vi "sine.vi"(7 "number of x points":i32=201, 8 "amplitude":dbl=1.0, 9 "phase":dbl, 10 "frequency":dbl=10000000.0, 11 "Sampling rate":i64=2000000000 format="%.0p") -> (1 "phase out (deg)":dbl[](array[numeric])=[0.0, 1.8000000000000003, 3.6000000000000005, 5.4, 7.200000000000001, 9.000000000000002, 10.8, 12.600000000000001, 14.400000000000002, 16.200000000000003, 18.000000000000004, 19.799999999999997, 21.6, 23.400000000000002, 25.200000000000003, 27.000000000000004, 28.800000000000004, 30.599999999999998, 32.400000000000006, 34.2, 36.00000000000001, 37.8, 39.599999999999994, 41.4, 43.2, 45.0, 46.800000000000004, 48.6, 50.400000000000006, 52.2, 54.00000000000001, 55.8, 57.60000000000001, 59.40000000000001, 61.199999999999996, 63.000000000000014, 64.80000000000001, 66.60000000000001, 68.4, 70.2, 72.00000000000001, 73.80000000000003, 75.6, 77.39999999999999, 79.19999999999999, 81.0, 82.8, 84.6, 86.4, 88.2, 90.0, 91.8, 93.60000000000001, 95.4, 97.2, 99.00000000000001, 100.80000000000001, 102.60000000000001, 104.4, 106.20000000000002, 108.00000000000001, 109.8, 111.6, 113.4, 115.20000000000002, 117.0, 118.80000000000003, 120.60000000000001, 122.39999999999999, 124.2, 126.00000000000003, 127.80000000000001, 129.60000000000002, 131.40000000000003, 133.20000000000002, 135.00000000000003, 136.8, 138.6, 140.4, 142.20000000000002, 144.00000000000003, 145.8, 147.60000000000005, 149.40000000000003, 151.2, 153.0, 154.79999999999998, 156.6, 158.39999999999998, 160.20000000000002, 162.0, 163.79999999999998, 165.6, 167.4, 169.2, 171.0, 172.8, 174.6, 176.4, 178.20000000000002, 180.0, 181.8, 183.6, 185.4, 187.20000000000002, 189.0, 190.8, 192.60000000000002, 194.4, 196.20000000000002, 198.00000000000003, 199.8, 201.60000000000002, 203.4, 205.20000000000002, 207.00000000000003, 208.8, 210.6, 212.40000000000003, 214.20000000000002, 216.00000000000003, 217.80000000000004, 219.6, 221.40000000000003, 223.2, 225.00000000000003, 226.8, 228.60000000000002, 230.40000000000003, 232.2, 234.0, 235.8, 237.60000000000005, 239.4, 241.20000000000002, 243.0, 244.79999999999998, 246.59999999999997, 248.4, 250.20000000000002, 252.00000000000006, 253.79999999999998, 255.60000000000002, 257.40000000000003, 259.20000000000005, 261.0, 262.80000000000007, 264.6, 266.40000000000003, 268.20000000000005, 270.00000000000006, 271.8, 273.6, 275.40000000000003, 277.2, 279.0, 280.8, 282.6, 284.40000000000003, 286.2, 288.00000000000006, 289.8, 291.6, 293.4, 295.2000000000001, 297.0, 298.80000000000007, 300.6, 302.4, 304.2, 306.0, 307.80000000000007, 309.59999999999997, 311.40000000000003, 313.2, 315.0, 316.79999999999995, 318.6, 320.40000000000003, 322.20000000000005, 324.0, 325.8, 327.59999999999997, 329.4, 331.2, 333.00000000000006, 334.8, 336.6, 338.4, 340.2, 342.0, 343.80000000000007, 345.6, 347.4, 349.2, 351.00000000000006, 352.8, 354.6, 356.40000000000003, 358.2, 0.0], 2 "y":dbl[](array[numeric])=[0.0, 0.03141075907812829, 0.06279051952931337, 0.09410831331851431, 0.12533323356430426, 0.1564344650402309, 0.1873813145857246, 0.21814324139654254, 0.2486898871648548, 0.2789911060392293, 0.30901699437494745, 0.33873792024529137, 0.3681245526846779, 0.3971478906347806, 0.42577929156507266, 0.4539904997395468, 0.4817536741017153, 0.5090414157503712, 0.5358267949789967, 0.5620833778521306, 0.5877852522924732, 0.6129070536529764, 0.6374239897486896, 0.6613118653236518, 0.6845471059286886, 0.7071067811865476, 0.7289686274214116, 0.7501110696304596, 0.7705132427757893, 0.7901550123756904, 0.8090169943749475, 0.8270805742745618, 0.8443279255020151, 0.8607420270039436, 0.8763066800438636, 0.8910065241883679, 0.9048270524660196, 0.9177546256839811, 0.9297764858882515, 0.9408807689542256, 0.9510565162951536, 0.9602936856769432, 0.9685831611286311, 0.9759167619387473, 0.9822872507286886, 0.9876883405951378, 0.9921147013144779, 0.99556196460308, 0.9980267284282716, 0.9995065603657316, 1.0, 0.9995065603657316, 0.9980267284282716, 0.99556196460308, 0.9921147013144778, 0.9876883405951378, 0.9822872507286887, 0.9759167619387474, 0.9685831611286311, 0.9602936856769431, 0.9510565162951535, 0.9408807689542255, 0.9297764858882515, 0.9177546256839811, 0.9048270524660195, 0.8910065241883679, 0.8763066800438635, 0.8607420270039436, 0.8443279255020152, 0.8270805742745617, 0.8090169943749472, 0.7901550123756903, 0.7705132427757893, 0.7501110696304594, 0.7289686274214114, 0.7071067811865472, 0.6845471059286885, 0.6613118653236518, 0.6374239897486895, 0.6129070536529764, 0.5877852522924728, 0.5620833778521305, 0.5358267949789962, 0.5090414157503711, 0.4817536741017156, 0.45399049973954686, 0.4257792915650729, 0.3971478906347806, 0.36812455268467814, 0.3387379202452913, 0.3090169943749475, 0.27899110603922955, 0.24868988716485482, 0.21814324139654276, 0.18738131458572457, 0.15643446504023098, 0.12533323356430454, 0.09410831331851435, 0.06279051952931358, 0.031410759078128236, 1.2246467991473532e-16, -0.03141075907812844, -0.06279051952931335, -0.0941083133185141, -0.12533323356430429, -0.15643446504023073, -0.18738131458572477, -0.2181432413965425, -0.24868988716485502, -0.2789911060392293, -0.3090169943749473, -0.3387379202452915, -0.3681245526846779, -0.3971478906347808, -0.42577929156507266, -0.4539904997395471, -0.4817536741017154, -0.5090414157503712, -0.5358267949789968, -0.5620833778521306, -0.5877852522924734, -0.6129070536529766, -0.6374239897486896, -0.661311865323652, -0.6845471059286887, -0.7071067811865477, -0.7289686274214116, -0.7501110696304598, -0.7705132427757894, -0.7901550123756904, -0.8090169943749473, -0.8270805742745616, -0.8443279255020153, -0.8607420270039438, -0.8763066800438636, -0.8910065241883678, -0.9048270524660194, -0.9177546256839809, -0.9297764858882515, -0.9408807689542255, -0.9510565162951538, -0.960293685676943, -0.9685831611286312, -0.9759167619387474, -0.9822872507286887, -0.9876883405951377, -0.9921147013144779, -0.99556196460308, -0.9980267284282716, -0.9995065603657316, -1.0, -0.9995065603657316, -0.9980267284282716, -0.99556196460308, -0.9921147013144779, -0.9876883405951378, -0.9822872507286886, -0.9759167619387473, -0.9685831611286311, -0.9602936856769431, -0.9510565162951533, -0.9408807689542256, -0.9297764858882512, -0.917754625683981, -0.9048270524660191, -0.891006524188368, -0.8763066800438634, -0.8607420270039434, -0.8443279255020155, -0.8270805742745618, -0.8090169943749476, -0.7901550123756901, -0.7705132427757896, -0.7501110696304595, -0.7289686274214116, -0.7071067811865477, -0.684547105928689, -0.6613118653236516, -0.6374239897486896, -0.6129070536529765, -0.5877852522924734, -0.5620833778521301, -0.5358267949789971, -0.5090414157503712, -0.4817536741017153, -0.4539904997395462, -0.425779291565073, -0.39714789063478034, -0.36812455268467786, -0.3387379202452914, -0.3090169943749477, -0.2789911060392288, -0.24868988716485535, -0.21814324139654243, -0.18738131458572468, -0.15643446504023023, -0.12533323356430465, -0.09410831331851403, -0.06279051952931326, -0.03141075907812836, -2.4492935982947064e-16], 3 "x":dbl[](array[numeric])=[0.0, 1.0, 2.0, 3.0, 4.0, 5.0, 6.0, 7.0, 8.0, 9.0, 10.0, 11.0, 12.0, 13.0, 14.0, 15.0, 16.0, 17.0, 18.0, 19.0, 20.0, 21.0, 22.0, 23.0, 24.0, 25.0, 26.0, 27.0, 28.0, 29.0, 30.0, 31.0, 32.0, 33.0, 34.0, 35.0, 36.0, 37.0, 38.0, 39.0, 40.0, 41.0, 42.0, 43.0, 44.0, 45.0, 46.0, 47.0, 48.0, 49.0, 50.0, 51.0, 52.0, 53.0, 54.0, 55.0, 56.0, 57.0, 58.0, 59.0, 60.0, 61.0, 62.0, 63.0, 64.0, 65.0, 66.0, 67.0, 68.0, 69.0, 70.0, 71.0, 72.0, 73.0, 74.0, 75.0, 76.0, 77.0, 78.0, 79.0, 80.0, 81.0, 82.0, 83.0, 84.0, 85.0, 86.0, 87.0, 88.0, 89.0, 90.0, 91.0, 92.0, 93.0, 94.0, 95.0, 96.0, 97.0, 98.0, 99.0, 100.0, 101.0, 102.0, 103.0, 104.0, 105.0, 106.0, 107.0, 108.0, 109.0, 110.0, 111.0, 112.0, 113.0, 114.0, 115.0, 116.0, 117.0, 118.0, 119.0, 120.0, 121.0, 122.0, 123.0, 124.0, 125.0, 126.0, 127.0, 128.0, 129.0, 130.0, 131.0, 132.0, 133.0, 134.0, 135.0, 136.0, 137.0, 138.0, 139.0, 140.0, 141.0, 142.0, 143.0, 144.0, 145.0, 146.0, 147.0, 148.0, 149.0, 150.0, 151.0, 152.0, 153.0, 154.0, 155.0, 156.0, 157.0, 158.0, 159.0, 160.0, 161.0, 162.0, 163.0, 164.0, 165.0, 166.0, 167.0, 168.0, 169.0, 170.0, 171.0, 172.0, 173.0, 174.0, 175.0, 176.0, 177.0, 178.0, 179.0, 180.0, 181.0, 182.0, 183.0, 184.0, 185.0, 186.0, 187.0, 188.0, 189.0, 190.0, 191.0, 192.0, 193.0, 194.0, 195.0, 196.0, 197.0, 198.0, 199.0, 200.0])   [LabVIEW 2017]
panel:
  out "Phase":dbl[](graph)=[0.0, 1.8000000000000003, 3.6000000000000005, 5.4, 7.200000000000001, 9.000000000000002, 10.8, 12.600000000000001, 14.400000000000002, 16.200000000000003, 18.000000000000004, 19.799999999999997, 21.6, 23.400000000000002, 25.200000000000003, 27.000000000000004, 28.800000000000004, 30.599999999999998, 32.400000000000006, 34.2, 36.00000000000001, 37.8, 39.599999999999994, 41.4, 43.2, 45.0, 46.800000000000004, 48.6, 50.400000000000006, 52.2, 54.00000000000001, 55.8, 57.60000000000001, 59.40000000000001, 61.199999999999996, 63.000000000000014, 64.80000000000001, 66.60000000000001, 68.4, 70.2, 72.00000000000001, 73.80000000000003, 75.6, 77.39999999999999, 79.19999999999999, 81.0, 82.8, 84.6, 86.4, 88.2, 90.0, 91.8, 93.60000000000001, 95.4, 97.2, 99.00000000000001, 100.80000000000001, 102.60000000000001, 104.4, 106.20000000000002, 108.00000000000001, 109.8, 111.6, 113.4, 115.20000000000002, 117.0, 118.80000000000003, 120.60000000000001, 122.39999999999999, 124.2, 126.00000000000003, 127.80000000000001, 129.60000000000002, 131.40000000000003, 133.20000000000002, 135.00000000000003, 136.8, 138.6, 140.4, 142.20000000000002, 144.00000000000003, 145.8, 147.60000000000005, 149.40000000000003, 151.2, 153.0, 154.79999999999998, 156.6, 158.39999999999998, 160.20000000000002, 162.0, 163.79999999999998, 165.6, 167.4, 169.2, 171.0, 172.8, 174.6, 176.4, 178.20000000000002, 180.0, 181.8, 183.6, 185.4, 187.20000000000002, 189.0, 190.8, 192.60000000000002, 194.4, 196.20000000000002, 198.00000000000003, 199.8, 201.60000000000002, 203.4, 205.20000000000002, 207.00000000000003, 208.8, 210.6, 212.40000000000003, 214.20000000000002, 216.00000000000003, 217.80000000000004, 219.6, 221.40000000000003, 223.2, 225.00000000000003, 226.8, 228.60000000000002, 230.40000000000003, 232.2, 234.0, 235.8, 237.60000000000005, 239.4, 241.20000000000002, 243.0, 244.79999999999998, 246.59999999999997, 248.4, 250.20000000000002, 252.00000000000006, 253.79999999999998, 255.60000000000002, 257.40000000000003, 259.20000000000005, 261.0, 262.80000000000007, 264.6, 266.40000000000003, 268.20000000000005, 270.00000000000006, 271.8, 273.6, 275.40000000000003, 277.2, 279.0, 280.8, 282.6, 284.40000000000003, 286.2, 288.00000000000006, 289.8, 291.6, 293.4, 295.2000000000001, 297.0, 298.80000000000007, 300.6, 302.4, 304.2, 306.0, 307.80000000000007, 309.59999999999997, 311.40000000000003, 313.2, 315.0, 316.79999999999995, 318.6, 320.40000000000003, 322.20000000000005, 324.0, 325.8, 327.59999999999997, 329.4, 331.2, 333.00000000000006, 334.8, 336.6, 338.4, 340.2, 342.0, 343.80000000000007, 345.6, 347.4, 349.2, 351.00000000000006, 352.8, 354.6, 356.40000000000003, 358.2, 0.0]
  out "Amplitude":dbl[](graph)=[0.0, 0.03141075907812829, 0.06279051952931337, 0.09410831331851431, 0.12533323356430426, 0.1564344650402309, 0.1873813145857246, 0.21814324139654254, 0.2486898871648548, 0.2789911060392293, 0.30901699437494745, 0.33873792024529137, 0.3681245526846779, 0.3971478906347806, 0.42577929156507266, 0.4539904997395468, 0.4817536741017153, 0.5090414157503712, 0.5358267949789967, 0.5620833778521306, 0.5877852522924732, 0.6129070536529764, 0.6374239897486896, 0.6613118653236518, 0.6845471059286886, 0.7071067811865476, 0.7289686274214116, 0.7501110696304596, 0.7705132427757893, 0.7901550123756904, 0.8090169943749475, 0.8270805742745618, 0.8443279255020151, 0.8607420270039436, 0.8763066800438636, 0.8910065241883679, 0.9048270524660196, 0.9177546256839811, 0.9297764858882515, 0.9408807689542256, 0.9510565162951536, 0.9602936856769432, 0.9685831611286311, 0.9759167619387473, 0.9822872507286886, 0.9876883405951378, 0.9921147013144779, 0.99556196460308, 0.9980267284282716, 0.9995065603657316, 1.0, 0.9995065603657316, 0.9980267284282716, 0.99556196460308, 0.9921147013144778, 0.9876883405951378, 0.9822872507286887, 0.9759167619387474, 0.9685831611286311, 0.9602936856769431, 0.9510565162951535, 0.9408807689542255, 0.9297764858882515, 0.9177546256839811, 0.9048270524660195, 0.8910065241883679, 0.8763066800438635, 0.8607420270039436, 0.8443279255020152, 0.8270805742745617, 0.8090169943749472, 0.7901550123756903, 0.7705132427757893, 0.7501110696304594, 0.7289686274214114, 0.7071067811865472, 0.6845471059286885, 0.6613118653236518, 0.6374239897486895, 0.6129070536529764, 0.5877852522924728, 0.5620833778521305, 0.5358267949789962, 0.5090414157503711, 0.4817536741017156, 0.45399049973954686, 0.4257792915650729, 0.3971478906347806, 0.36812455268467814, 0.3387379202452913, 0.3090169943749475, 0.27899110603922955, 0.24868988716485482, 0.21814324139654276, 0.18738131458572457, 0.15643446504023098, 0.12533323356430454, 0.09410831331851435, 0.06279051952931358, 0.031410759078128236, 1.2246467991473532e-16, -0.03141075907812844, -0.06279051952931335, -0.0941083133185141, -0.12533323356430429, -0.15643446504023073, -0.18738131458572477, -0.2181432413965425, -0.24868988716485502, -0.2789911060392293, -0.3090169943749473, -0.3387379202452915, -0.3681245526846779, -0.3971478906347808, -0.42577929156507266, -0.4539904997395471, -0.4817536741017154, -0.5090414157503712, -0.5358267949789968, -0.5620833778521306, -0.5877852522924734, -0.6129070536529766, -0.6374239897486896, -0.661311865323652, -0.6845471059286887, -0.7071067811865477, -0.7289686274214116, -0.7501110696304598, -0.7705132427757894, -0.7901550123756904, -0.8090169943749473, -0.8270805742745616, -0.8443279255020153, -0.8607420270039438, -0.8763066800438636, -0.8910065241883678, -0.9048270524660194, -0.9177546256839809, -0.9297764858882515, -0.9408807689542255, -0.9510565162951538, -0.960293685676943, -0.9685831611286312, -0.9759167619387474, -0.9822872507286887, -0.9876883405951377, -0.9921147013144779, -0.99556196460308, -0.9980267284282716, -0.9995065603657316, -1.0, -0.9995065603657316, -0.9980267284282716, -0.99556196460308, -0.9921147013144779, -0.9876883405951378, -0.9822872507286886, -0.9759167619387473, -0.9685831611286311, -0.9602936856769431, -0.9510565162951533, -0.9408807689542256, -0.9297764858882512, -0.917754625683981, -0.9048270524660191, -0.891006524188368, -0.8763066800438634, -0.8607420270039434, -0.8443279255020155, -0.8270805742745618, -0.8090169943749476, -0.7901550123756901, -0.7705132427757896, -0.7501110696304595, -0.7289686274214116, -0.7071067811865477, -0.684547105928689, -0.6613118653236516, -0.6374239897486896, -0.6129070536529765, -0.5877852522924734, -0.5620833778521301, -0.5358267949789971, -0.5090414157503712, -0.4817536741017153, -0.4539904997395462, -0.425779291565073, -0.39714789063478034, -0.36812455268467786, -0.3387379202452914, -0.3090169943749477, -0.2789911060392288, -0.24868988716485535, -0.21814324139654243, -0.18738131458572468, -0.15643446504023023, -0.12533323356430465, -0.09410831331851403, -0.06279051952931326, -0.03141075907812836, -2.4492935982947064e-16]
  # "2019/06/27 NT"
  # "y = a*sin(2*pi*b*x +c)     sine wave"
  # "Run twice to see full curve (program logic - doesn't affect array)"
  # "(b)"
  # "(c)"
  # "(a)"
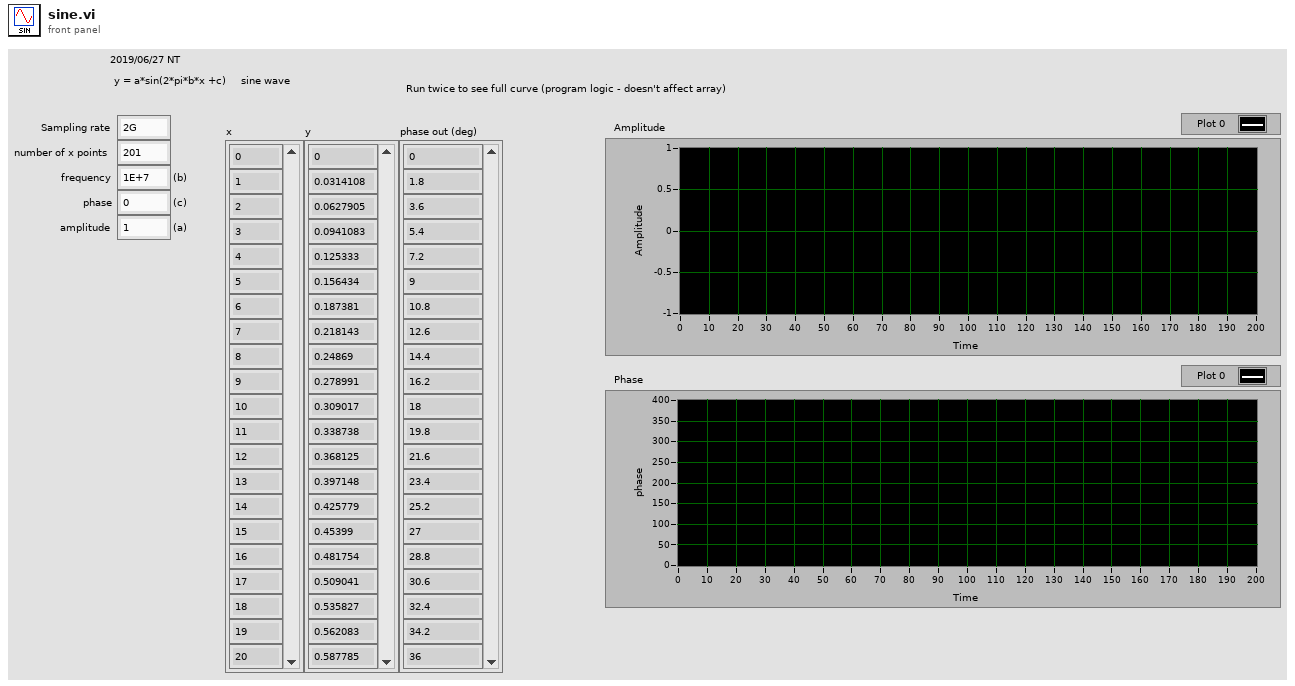
[diagram p1: front panel]
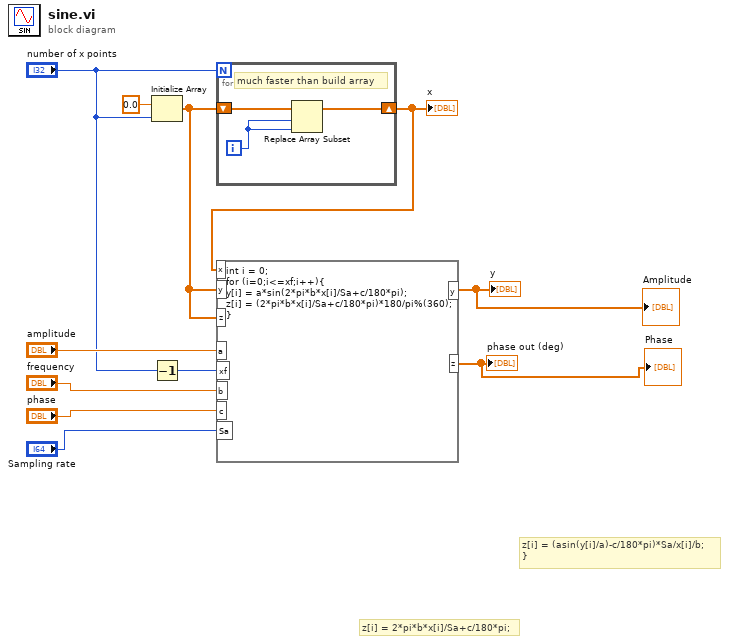
[diagram p0: block diagram]
diagram:
  # "z[i] = 2*pi*b*x[i]/Sa+c/180*pi;"
  # "z[i] = (asin(y[i]/a)-c/180*pi)*Sa/x[i]/b;\n}"
  n1 = Initialize Array(0.0 ("element"), "number of x points") -> (w2:dbl[])
  n2 = Decrement(x="number of x points") -> (x-1=w9:i32)
  n3 = for {
    N: "number of x points" -> [_]
    shift-right: [w13] -> w6
    shift-left: w2 -> [w14]
    i -> [w12]
    # "much faster than build array"
    n4 = Replace Array Subset(array=w14, new element=w12, index=w12) -> (w13:dbl[])
  }
  "x" <- w6
  n5 = formula code="int i = 0;\nfor (i=0;i<=xf;i++){\ny[i] = a*sin(2*pi*b*x[i]/Sa+c/180*pi);\nz[i] = (2*pi*b*x[i]/Sa+c/180*pi)*180/pi%(360);\n}"("x"=w6, "y"=w2, "a"="amplitude", "xf"=w9, "b"="frequency", "c"="phase", "Sa"="Sampling rate", "z"=w2) -> ("y"=→"y" →"Amplitude":dbl[], "z"=→"phase out (deg)" →"Phase":dbl[])
